vi "Global_CMD to SM Data.vi"() -> ()   [LabVIEW 2017, in "Intake.lvlib"]
uses:
  Intake.lvlib
  Cluster_Cmd to SM Data.ctl
  Enum_SM Cmd Select.ctl
panel:
  in  "Cmd_Intake":T1
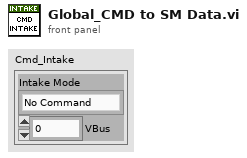
[diagram p1: front panel]
types:
  T1 = typedef "Intake.lvlib/Cluster_Cmd to SM Data.ctl" = cluster{"Intake Mode":T2, "VBus":dbl}
  T2 = typedef "Intake.lvlib/Enum_SM Cmd Select.ctl" = enum16{"No Command", "Manual", "Half Speed", "Full Speed", "Reverse", "Stop"}
diagram:
